vi "save_increment.vi"(8 "error in (no error)":errorcluster, 11 "HGF_Reference":refnum<class "HGF_Reference.lvclass">) -> (0 "error out":errorcluster, 3 "dup HGF_Reference":refnum<class "HGF_Reference.lvclass">)   [LabVIEW 2009, in "HB_BaseClass_Examples.lvlib" / "HB_Simple.lvclass"]
doc: "This VI provides a method to increment the referenced object attribute with giving direct access to it wire."
uses:
  HB_Simple.lvclass
  lib.lib/HGF_LVC/HGF_BaseClasses/HGF_Reference/HGF_Reference.lvclass
panel:
  in  "timeout in ms (-1)":i32=-1
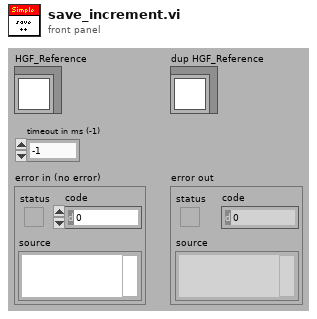
[diagram p1: front panel]
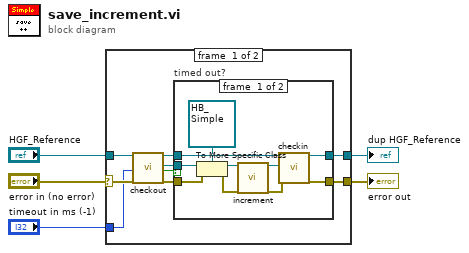
[diagram p0: block diagram]
diagram:
  n1 = case shown="No Error" "error in (no error)" {
    selector: "error in (no error)" -> [w8 w28]
    tunnel: [w7 w28] -> w4
    tunnel: [w10 w27] -> w2
    tunnel: "HGF_Reference" -> [w11 w27]
    tunnel: "timeout in ms (-1)" -> [w6 _]
    frame #0 {
      n2 = call "checkout.vi"("HGF_Reference"=w11, "timeout in ms (-1)"=w6, "error in (no error)"=w8) -> ("dup HGF_Reference"=w14:refnum<class "HGF_Reference.lvclass">, "Object"=w12:refnum<class>, "got object?"=w9:bool, "error out"=w13:errorcluster)  [unwired: 13 out]
      n3 = case "timed out?" shown="False" w9 {
        tunnel: w14 -> [w24 w26]
        tunnel: w13 -> [w23 w25]
        tunnel: w12 -> [w22 _]
        tunnel: [w16 w26] -> w10
        tunnel: [w15 w25] -> w7
        frame #0 {
          n4 = To More Specific Class(target class=refnum<class "HB_Simple.lvclass"> refnum ("HB_Simple in"), reference=w22, error in=w23) -> (specific class reference=w21:refnum<class "HB_Simple.lvclass">, error out=w19:errorcluster)
          n5 = call "increment.vi"("HB_Simple in"=w21, "error in (no error)"=w19) -> ("HB_Simple out"=w20:refnum<class "HB_Simple.lvclass">, "error out"=w18:errorcluster)  [unwired: 16 out]
          n6 = call "checkin.vi"("HGF_Reference"=w24, "Object"=w20, "error in (no error)"=w18) -> ("dup HGF_Reference"=w16:refnum<class "HGF_Reference.lvclass">, "error out"=w15:errorcluster)  [unwired: 1 in, 14 out]
        }
        frame #1 {
        }
      }
    }
    frame #1 {
    }
  }
  "error out" <- w4
  "dup HGF_Reference" <- w2
